vi "Array Level Estimation.vi"(8 "Error In":errorcluster, 9 "Method (Mode)":T1, 11 "Array":dbl[](array[numeric])) -> (0 "Error Out":errorcluster, 3 "Level":dbl)   [LabVIEW 2021, in "Arrays.lvlib"]
doc: "Find mode (or mean) of an array by computing it for increasingly fine-grained histograms of the array and returning the average value."
uses:
  Arrays.lvlib
  Fits/Square Pulse/Square Pulse Levels Type.ctl
  Histograms/Histogram Bin Option.ctl
  Histograms/Linear Histogram Options.ctl
  Histograms/Histogram Bin Position.ctl
  9f7114d6-7e51-4058-b29f-ee62147b84b6.vi
  9f7114d6-7e51-4058-b29f-ee62147b84b6.vi/b1828c6e-eb0a-43e9-a724-8b596c52e435.vi
  9f7114d6-7e51-4058-b29f-ee62147b84b6.vi/7a6138ed-c001-4311-b538-9ba42ae7c7b1.vi
  9f7114d6-7e51-4058-b29f-ee62147b84b6.vi/52c6b4fa-501b-4af0-803b-8bab516ca5d3.vi
  9f7114d6-7e51-4058-b29f-ee62147b84b6.vi/d7237e10-35ab-4bcb-a0c6-4883c3f4c990.vi
  9f7114d6-7e51-4058-b29f-ee62147b84b6.vi/5fb5dd96-3b97-4592-ba56-58181c8e7105.vi
  9f7114d6-7e51-4058-b29f-ee62147b84b6.vi/8e13a849-a393-4484-9968-4af7b25c38d7.vi
  Time/High Resolution Timing.vi
  <userlib>/_OpenG.lib/array/array.llb/Filter 1D Array__ogtk.vi
  <userlib>/_OpenG.lib/array/array.llb/Filter 1D Array (DBL)__ogtk.vi
  <userlib>/_OpenG.lib/array/array.llb/Delete Elements from Array__ogtk.vi
  <userlib>/_OpenG.lib/array/array.llb/Delete Elements from 1D Array (DBL)__ogtk.vi
  <vilib>/Utility/error.llb/Error Cluster From Error Code.vi
  Histograms/Histogram Window.lvlib
  Utilities/Utilities.lvlib
  Fits/Fits.lvlib
panel:
  out "XY Graph":cluster{i32[], dbl[]}[](graph)
  # "see the AlliGator License on the block diagram (Ctrl+E or Window:Show Block Diagram)"
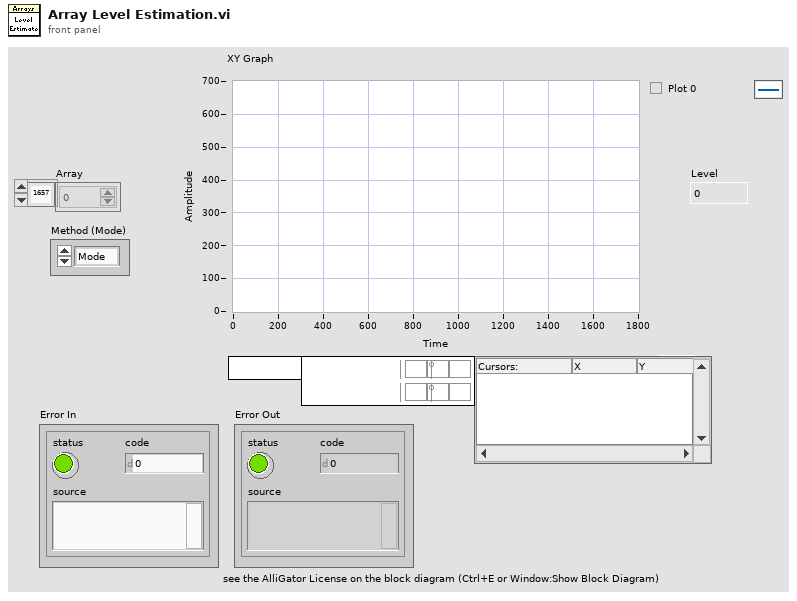
[diagram p1: front panel]
types:
  T1 = typedef "Fits.lvlib/Square Pulse Levels Type.ctl" = enum16{"Mode", "Mean"}
  T2 = typedef "Histogram Window.lvlib/Histogram Bin Option.ctl" = enum32{"Bin Number", "Bin Size"}
  T3 = typedef "Histogram Window.lvlib/Linear Histogram Options.ctl" = cluster{"Bin Size":dbl, "Bin Number":i32, "Bin Option":T2, "Min Value":dbl, "Max Value":dbl, "Filter NaN & Infinite Values":bool, "Frequency Plot":bool, "Align Bins":bool, "Bin Location":T4, "Project Outside Values":bool, "Max Histogram Size":i32}
  T4 = typedef "Histogram Window.lvlib/Histogram Bin Position.ctl" = enum16{"Left", "Center", "Right"}
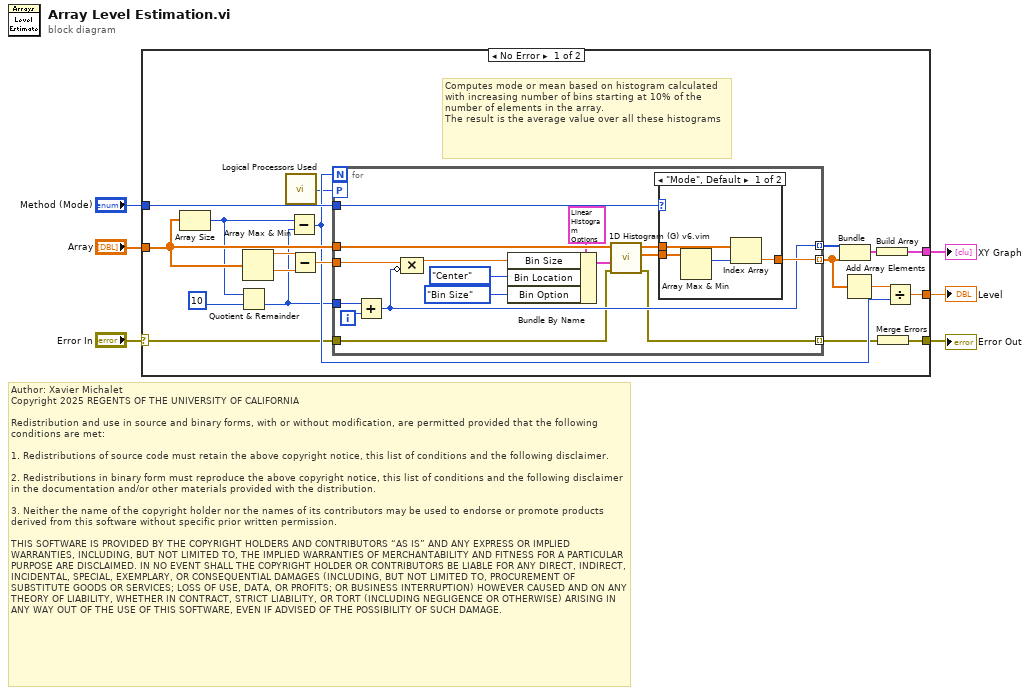
[diagram p0: block diagram]
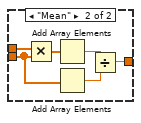
[diagram p2: hidden frame]
diagram:
  # "Author: Xavier Michalet\nCopyright 2025 REGENTS OF THE UNIVERSITY OF CALIFORNIA\n\nRedistribution and use in source and binary forms, with or without modification, are permitted provided that the following conditions are met:\n\n1. Redistributions of source code must retain the above copyright notice, this list of conditions and the following disclaimer.\n\n2. Redistributions in binary form must reproduce the above copyright notice, this list of conditions and the following disclaimer in the documentation and/or other materials provided with the distribution.\n\n3. Neither the name of the copyright holder nor the names of its contributors may be used to endorse or promote products derived from this software without specific prior written permission.\n\nTHIS SOFTWARE IS PROVIDED BY THE COPYRIGHT HOLDERS AND CONTRIBUTORS “AS IS” AND ANY EXPRESS OR IMPLIED WARRANTIES, INCLUDING, BUT NOT LIMITED TO, THE IMPLIED WARRANTIES OF MERCHANTABILITY AND FITNESS FOR A PARTICULAR PURPOSE ARE DISCLAIMED. IN NO EVENT SHALL THE COPYRIGHT HOLDER OR CONTRIBUTORS BE LIABLE FOR ANY DIRECT, INDIRECT, INCIDENTAL, SPECIAL, EXEMPLARY, OR CONSEQUENTIAL DAMAGES (INCLUDING, BUT NOT LIMITED TO, PROCUREMENT OF SUBSTITUTE GOODS OR SERVICES; LOSS OF USE, DATA, OR PROFITS; OR BUSINESS INTERRUPTION) HOWEVER CAUSED AND ON ANY THEORY OF LIABILITY, WHETHER IN CONTRACT, STRICT LIABILITY, OR TORT (INCLUDING NEGLIGENCE OR OTHERWISE) ARISING IN ANY WAY OUT OF THE USE OF THIS SOFTWARE, EVEN IF ADVISED OF THE POSSIBILITY OF SUCH DAMAGE."
  n1 = case shown="No Error" "Error In" {
    selector: "Error In" -> [w10 w52]
    tunnel: "Array" -> [w25 _]
    tunnel: "Method (Mode)" -> [w21 _]
    tunnel: [w18 _] -> w4
    tunnel: [w15 _] -> w3
    tunnel: [w8 w52] -> w1
    frame No Error {
      # "Computes mode or mean based on histogram calculated with increasing number of bins starting at 10% of the number of elements in the array.\nThe result is the average value over all these histograms"
      n2 = Array Size(array=w25) -> (size(s)=w14:i32)
      n3 = Quotient & Remainder(x=w14, y=10 ("size(s)")) -> (floor(x/y)=w11:i32)  [unwired: 1 out]
      n4 = Array Max & Min(array=w25) -> (max value=w24:dbl, min value=w23:dbl)  [unwired: 2 out]
      n5 = call "Logical Processors Used.vi"() -> ("# Logical Processor Used"=w7:i32)  [unwired: 6 in]
      n6 = Subtract(x=w14, y=w11) -> (x-y=w12:i32)
      n7 = Subtract(x=w24, y=w23) -> (x-y=w22:dbl)
      n8 = for {
        N: w12 -> [_]
        tunnel: w25 -> [w41]
        tunnel: w22 -> [w40]
        tunnel: w21 -> [w37]
        tunnel: [w36] -> w17 mode=indexing
        tunnel: [w35] -> w20 mode=indexing
        tunnel: w11 -> [w34]
        workers-P: w7 -> [_]
        tunnel: w10 -> [w32]
        tunnel: [w31] -> w9 mode=indexing
        i -> [w33]
        n9 = Add(x=w34, y=w33) -> (x+y=w35:i32)
        n10 = Compound Arithmetic op=MULTIPLY(w40, invert w35) -> (w28:dbl)
        n11 = Bundle By Name(cluster=T3 {"Bin Size"=nan, "Bin Number"=0, "Bin Option"=enum."Bin Number", "Min Value"=-inf, "Max Value"=inf, "Filter NaN & Infinite Values"=FALSE, "Frequency Plot"=FALSE, "Align Bins"=FALSE, "Bin Location"=enum."Left", "Project Outside Values"=FALSE, "Max Histogram Size"=100000} ("Histogram Options"), "Bin Size"=w28, "Bin Location"=Histogram_Bin_Position."Center" ("Bin Location (Left)"), "Bin Option"=Histogram_Bin_Option."Bin Size" ("Bin Size")) -> (w29:T3)
        n12 = call "1D Histogram (G) v6.vim"("Error In"=w32, "Histogram Options"=w29, "Array"=w41) -> ("Error Out"=w31:errorcluster, "Histogram"=w38:dbl[], "Axis"=w39:dbl[])  [unwired: 2 in, 4 out]
        n13 = case shown="\"Mode\", Default" w37 {
          tunnel: w38 -> [w45 w49]
          tunnel: w39 -> [w44 w51]
          tunnel: [w42 w46] -> w36
          frame "Mode", Default {
            n14 = Array Max & Min(array=w45) -> (max index (indices)=w43:i32)  [unwired: 3 out]
            n15 = Index Array(array=w44, index=w43) -> (element=w42:dbl)
          }
          frame "Mean" {
            n16 = Multiply(x=w51, y=w49) -> (x*y=w50:dbl[])
            n17 = Add Array Elements(numeric array=w50) -> (sum=w48:dbl)
            n18 = Add Array Elements(numeric array=w49) -> (sum=w47:dbl)
            n19 = Divide(x=w48, y=w47) -> (x/y=w46:dbl)
          }
        }
      }
      n20 = Bundle(w20, w17) -> (w19:cluster{i32[], dbl[]})  [unwired: 1 in]
      n21 = Add Array Elements(numeric array=w17) -> (sum=w16:dbl)
      n22 = Build Array(w19) -> (w18:cluster{i32[], dbl[]}[])
      n23 = Merge Errors(w9) -> (w8:errorcluster)
      n24 = Divide(x=w16, y=w12) -> (x/y=w15:dbl)
    }
    frame Error {
    }
  }
  "XY Graph" <- w4
  "Level" <- w3
  "Error Out" <- w1
